vi "FGV_Test_Class.vi"(0 "Action":T2(ring), 5 "Test":refnum<class "Test (Default).lvclass">, 7 "Test class":string, 9 "Test Name":string, 11 "error in (no error)":errorcluster, 12 "Parameter (Json) en entrée":string) -> (4 "Test (Default).lvclass":refnum<class "Test (Default).lvclass">, 6 "List Test":T1(array[cluster]), 14 "Parameter (Json) en sortie":string, 15 "error out":errorcluster)   [LabVIEW 2020, in "Library Commun.lvlib"]
uses:
  Library Commun.lvlib
  Class/Test/Test (Default)/Test (Default).lvclass
  Class/JSON API/Variant JSON/Variant to JSON.vi
  Class/JSON API/JSON Value/Get Item by name array.vi
  Class/JSON API/JSON Value/JSON Value.lvclass
  Class/JSON API/Get Polymorphic/JSON GetSet.lvlib
  Class/JSON API/Variant JSON/Variant JSON.lvlib
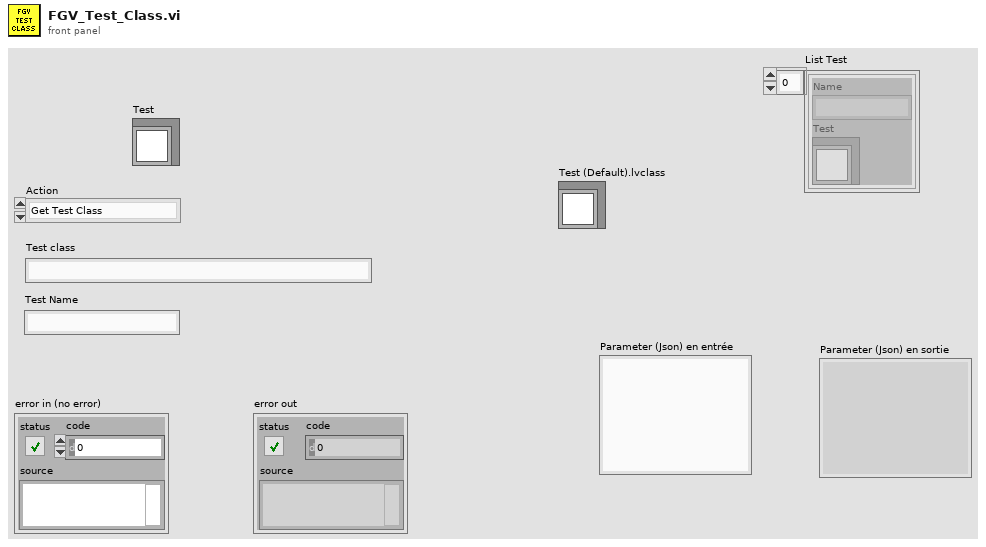
[diagram p1: front panel]
types:
  T1 = cluster{"Name":string, "Test":refnum<class "Test (Default).lvclass">}[]
  T2 = enum16{"Get Test Class", "Set Test object", "Get Test object", "List Test", "Init"}
  T3 = cluster{"Test Name":string, "Test":refnum<class "Test (Default).lvclass">}
  T4 = cluster{"Test Name":string, "Test":refnum<class "Test (Default).lvclass">}[]
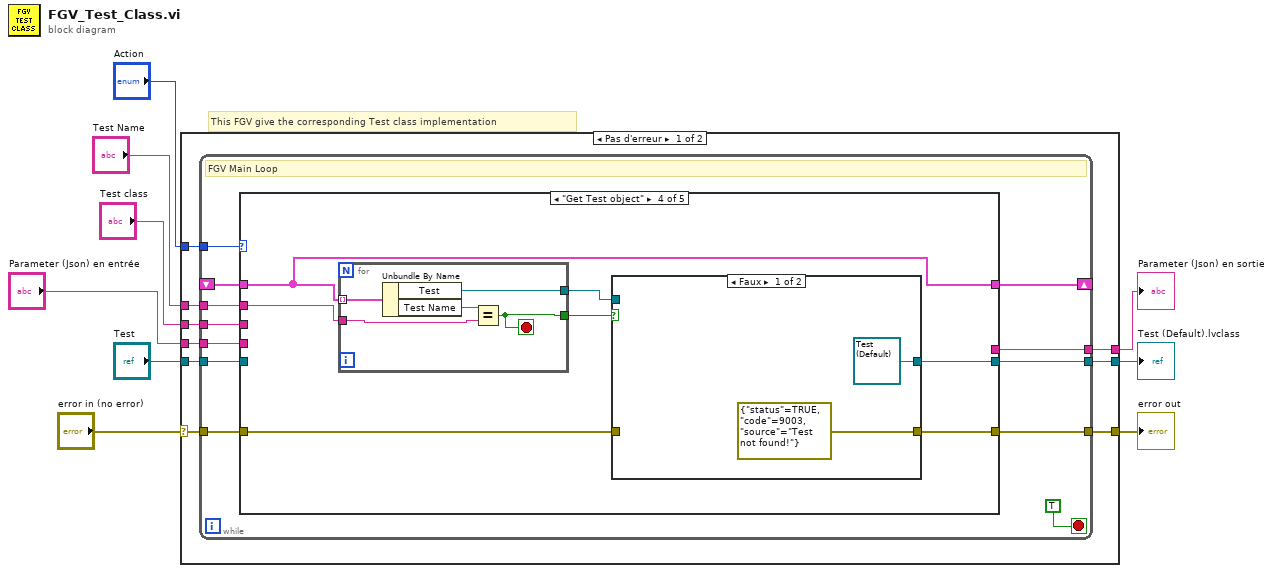
[diagram p0: block diagram]
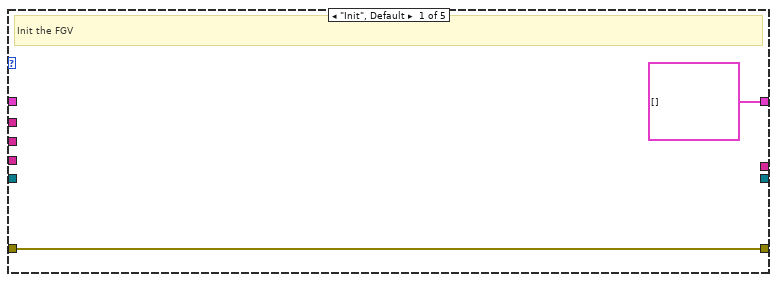
[diagram p2: hidden frame]
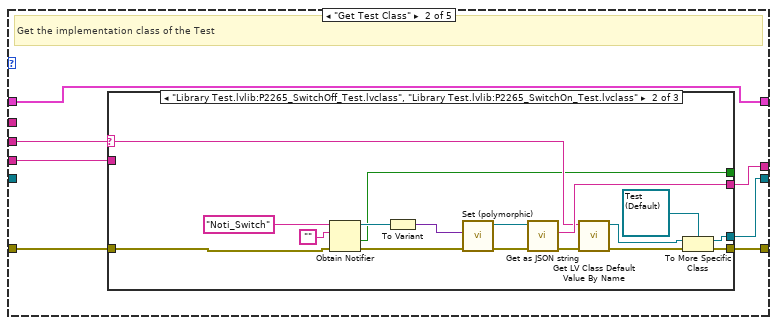
[diagram p3: hidden frame]
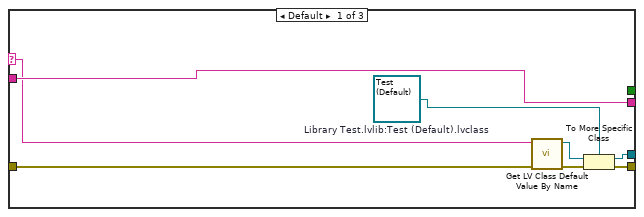
[diagram p4: hidden frame]
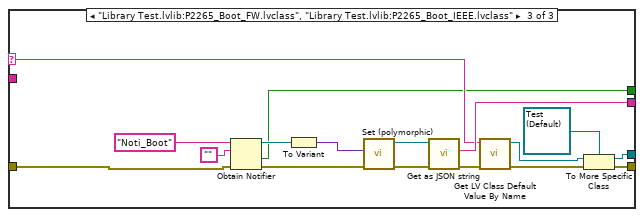
[diagram p5: hidden frame]
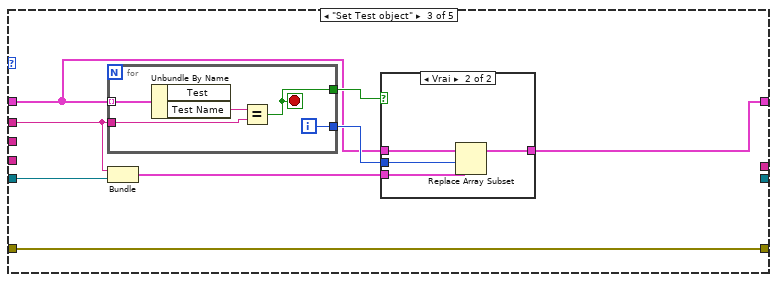
[diagram p6: hidden frame]
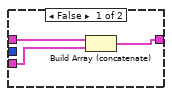
[diagram p7: hidden frame]
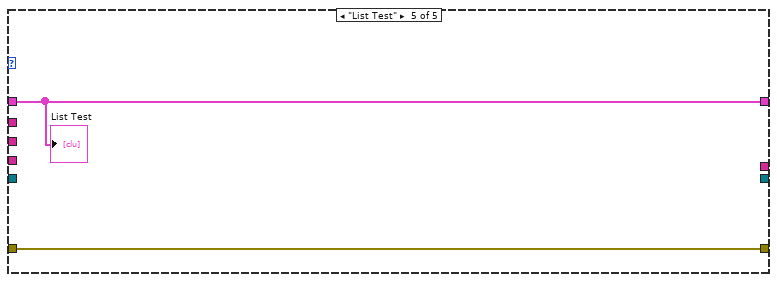
[diagram p9: hidden frame]
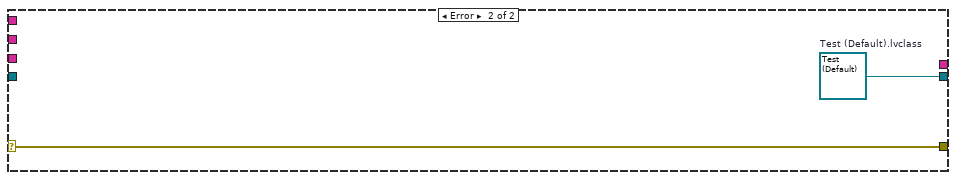
[diagram p10: hidden frame]
diagram:
  # "This FGV give the corresponding Test class implementation"
  n1 = case shown="Pas d'erreur" "error in (no error)" {
    selector: "error in (no error)" -> [w17 w121]
    tunnel: [w16 w121] -> w8
    tunnel: "Action" -> [w18 _]
    tunnel: "Test class" -> [w15 _]
    tunnel: [w14 w120] -> w5
    tunnel: [w13 _] -> w4
    tunnel: "Parameter (Json) en entrée" -> [w12 _]
    tunnel: "Test" -> [w11 _]
    tunnel: "Test Name" -> [w10 _]
    frame No Error {
      n2 = while {
        tunnel: w18 -> [w30]
        tunnel: w17 -> [w29]
        tunnel: [w28] -> w16
        tunnel: w15 -> [w27]
        tunnel: [w25] -> w14
        tunnel: [w24] -> w13
        tunnel: w12 -> [w23]
        shift-right: [w22] -> _
        shift-left: _ -> [w21]
        tunnel: w11 -> [w20]
        tunnel: w10 -> [w19]
        stop <- TRUE stop-if-true
        # "FGV Main Loop"
        n3 = case shown="\"Get Test object\"" w30 {
          tunnel: w29 -> [w32 w38 w89 w102 w118]
          tunnel: [w32 w37 w89 w103 w118] -> w28
          tunnel: w27 -> [_ w33 _ _ _]
          tunnel: [_ w39 _ w105 _] -> w25
          tunnel: [_ w36 _ _ _] -> w24
          tunnel: w23 -> [_ w35 _ _ _]
          tunnel: [T1 [] ("List Test") w34 w85 w107 w119] -> w22
          tunnel: w21 -> [_ w34 w86 w107 w119]
          tunnel: w20 -> [_ _ w84 _ _]
          tunnel: w19 -> [_ _ w83 w108 _]
          frame "Init", Default {
            # "Init the FGV"
          }
          frame "Get Test Class" {
            # "Get the implementation class of the Test"
            n4 = case shown="\"Library Test.lvlib:P2265_SwitchOff_Test.lvclass\", \"Library Test.lvlib:P2265_SwitchOn_Test.lvclass\"" w33 {
              selector: w33 -> [w40 w49 w66]
              tunnel: [w46 w61 w78] -> w39
              tunnel: w38 -> [w41 w59 w76]
              tunnel: [w45 w60 w77] -> w37
              tunnel: [w44 w52 w69] -> w36
              tunnel: w35 -> [w44 _ _]
              tunnel: [_ w48 w65] -> _
              frame Default {
                w47 = refnum<class "Test (Default).lvclass"> refnum  # Library Test.lvlib:Test (Default).lvclass
                n5 = call <vilib>:"Get LV Class Default Value By Name.vi"("error in (no error)"=w41, "class name"=w40) -> ("error out"=w43:errorcluster, "object"=w42:refnum<class>)  [unwired: 8 in]
                n6 = To More Specific Class(target class=w47, reference=w42, error in=w43) -> (specific class reference=w46:refnum<class "Test (Default).lvclass">, error out=w45:errorcluster)
              }
              frame "Library Test.lvlib:P2265_SwitchOff_Test.lvclass", "Library Test.lvlib:P2265_SwitchOn_Test.lvclass" {
                n7 = Obtain Notifier(name (unnamed)="Noti_Switch" ("class name"), notification data type="", error in (no error)=w59) -> (notifier out=w51:refnum<notifier>, created new?=w48:bool, error out=w54:errorcluster)  [unwired: 1 in]
                n8 = To Variant(anything=w51) -> (Variant=w57:variant)
                n9 = call-poly "Set (polymorphic).vi"("error in (no error)"=w54, "Variant"=w57) -> ("error out"=w55:errorcluster, "JSON Value out"=w56:refnum<class "JSON Value.lvclass">)  [unwired: 8 in]
                n10 = call "Get as JSON string.vi"("error in (no error)"=w55, "JSON Value in"=w56) -> ("error out"=w53:errorcluster, "<JSON>"=w52:string)  [unwired: 8 in]
                n11 = call <vilib>:"Get LV Class Default Value By Name.vi"("error in (no error)"=w53, "class name"=w49) -> ("error out"=w64:errorcluster, "object"=w63:refnum<class>)  [unwired: 8 in]
                n12 = To More Specific Class(target class=refnum<class "Test (Default).lvclass"> refnum ("Library Test.lvlib:Test (Default).lvclass"), reference=w63, error in=w64) -> (specific class reference=w61:refnum<class "Test (Default).lvclass">, error out=w60:errorcluster)
              }
              frame "Library Test.lvlib:P2265_Boot_FW.lvclass", "Library Test.lvlib:P2265_Boot_IEEE.lvclass" {
                n13 = Obtain Notifier(name (unnamed)="Noti_Boot" ("class name"), notification data type="", error in (no error)=w76) -> (notifier out=w68:refnum<notifier>, created new?=w65:bool, error out=w71:errorcluster)  [unwired: 1 in]
                n14 = To Variant(anything=w68) -> (Variant=w74:variant)
                n15 = call-poly "Set (polymorphic).vi"("error in (no error)"=w71, "Variant"=w74) -> ("error out"=w72:errorcluster, "JSON Value out"=w73:refnum<class "JSON Value.lvclass">)  [unwired: 8 in]
                n16 = call "Get as JSON string.vi"("error in (no error)"=w72, "JSON Value in"=w73) -> ("error out"=w70:errorcluster, "<JSON>"=w69:string)  [unwired: 8 in]
                n17 = call <vilib>:"Get LV Class Default Value By Name.vi"("error in (no error)"=w70, "class name"=w66) -> ("error out"=w81:errorcluster, "object"=w80:refnum<class>)  [unwired: 8 in]
                n18 = To More Specific Class(target class=refnum<class "Test (Default).lvclass"> refnum ("Library Test.lvlib:Test (Default).lvclass"), reference=w80, error in=w81) -> (specific class reference=w78:refnum<class "Test (Default).lvclass">, error out=w77:errorcluster)
              }
            }
          }
          frame "Set Test object" {
            n19 = for {
              tunnel: w86 -> [w101] mode=indexing
              tunnel: [w99] -> w88
              tunnel: [w98] -> w87
              tunnel: w83 -> [w97]
              i -> [w98]
              stop <- w99 stop-if-true
              n20 = Unbundle By Name(w101) -> ("Test Name"=w100:string)  [unwired: 1 out]
              n21 = Equal?(x=w100, y=w97) -> (x = y?=w99:bool)
            }
            n22 = Bundle("Test Name"=w83, "Test"=w84) -> (w82:T3)  [unwired: 1 in]
            n23 = case shown="Vrai" w88 {
              tunnel: [w92 w93] -> w85
              tunnel: w86 -> [w91 w96]
              tunnel: w82 -> [w90 w94]
              tunnel: w87 -> [_ w95]
              frame False {
                n24 = Build Array (concatenate)(w91, w90) -> (w92:T4)
              }
              frame True {
                n25 = Replace Array Subset(array=w96, new element=w94, index=w95) -> (w93:T4)
              }
            }
          }
          frame "Get Test object" {
            n26 = for {
              tunnel: w107 -> [w117] mode=indexing
              tunnel: w108 -> [w115]
              tunnel: [w114] -> w104
              tunnel: [w113] -> w106
              stop <- w113 stop-if-true
              n27 = Unbundle By Name(w117) -> ("Test"=w114:refnum<class "Test (Default).lvclass">, "Test Name"=w116:string)
              n28 = Equal?(x=w116, y=w115) -> (x = y?=w113:bool)
            }
            n29 = case shown="Faux" w106 {
              tunnel: [refnum<class "Test (Default).lvclass"> refnum ("Test") w112] -> w105
              tunnel: w104 -> [_ w112]
              tunnel: [errorcluster {"status"=TRUE, "code"=9003, "source"="Test not found!"} ("error constant") w111] -> w103
              tunnel: w102 -> [_ w111]
              frame False {
              }
              frame True {
              }
            }
          }
          frame "List Test" {
            "List Test" <- w119
          }
        }
      }
    }
    frame Error {
      w120 = refnum<class "Test (Default).lvclass"> refnum  # Test (Default).lvclass
    }
  }
  "error out" <- w8
  "Test (Default).lvclass" <- w5
  "Parameter (Json) en sortie" <- w4
